vi "FPGA_RefCurrGathering.vi"() -> ()   [LabVIEW 2014]
uses:
  <vilib>/rvi/Emulation/niFpgaGetClockAttributes.vi
  <vilib>/rvi/Emulation/niFpgaSctlEmulationGetInTimedLoop.vi
  <vilib>/rvi/Emulation/niFpgaEmulationReportErrorSimple.vi
  <vilib>/rvi/eio/common/nirviEmuTemplateMethod_errors.vi
  <vilib>/rvi/Emulation/niFpgaCriticalErrorInLSC.vi
  <vilib>/eio/EIONode/EIONode.xnode
panel:
  out "RefCurr":i16
  out "GatherFinished?":bool
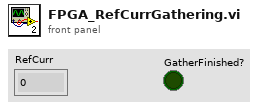
[diagram p1: front panel]
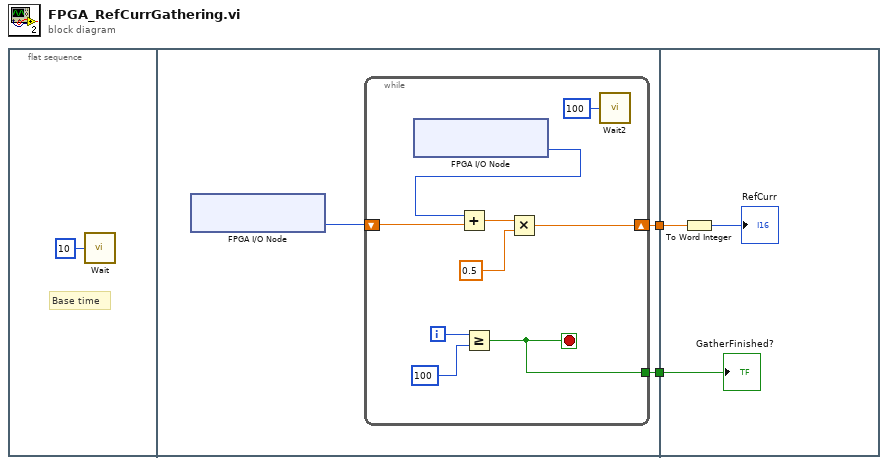
[diagram p0: block diagram]
diagram:
  n1 = flat-sequence {
    tunnel: [w5] -> w2
    tunnel: [w4] -> w1
    tunnel: w2 -> [w18]
    tunnel: w1 -> [w16]
    frame #0 {
      # "Base time"
      n2 = call "Wait"("Count(mSec)"=u32 10) -> ()  [unwired: 1 out]
    }
    frame #1 {
      n3 = xnode "FPGA I/O Node"() -> ("Connector0/AI1"=w6:i16)  [unwired: 1 in, 1 out]
      n4 = while {
        shift-right: [w11] -> w5
        shift-left: w6 -> [w15]
        tunnel: [w7] -> w4
        i -> [w9]
        stop <- w7 stop-if-true
        n5 = xnode "FPGA I/O Node"() -> ("Connector0/AI1"=w14:i16)  [unwired: 1 in, 1 out]
        n6 = Add(x=w14, y=w15) -> (x+y=w13:sgl)
        n7 = Greater Or Equal?(x=w9, y=100) -> (x >= y?=w7:bool)
        n8 = Multiply(x=w13, y=sgl 0.5) -> (x*y=w11:sgl)
        n9 = call "Wait2"("Count(uSec)"=u32 100) -> ()  [unwired: 1 out]
      }
    }
    frame #2 {
      n10 = To Word Integer(number=w18) -> (16bit integer=→"RefCurr":i16)
      "GatherFinished?" <- w16
    }
  }
